vi "仁科遥控对话框.vi"() -> ()   [LabVIEW 2016, in "环境动力监测库.lvlib" / "空调库.lvlib"]
panel:
  in  "关机发射":bool
  in  "开机制热发射":bool
  in  "开机制冷发射":bool
  in  "关机学习":bool
  in  "开机制热学习":bool
  in  "开机制冷学习":bool
  # "学习遥控器"
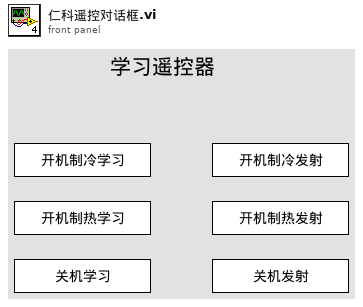
[diagram p1: front panel]
types:
  T1 = enum16{"open", "read", "write single", "write", "close"}
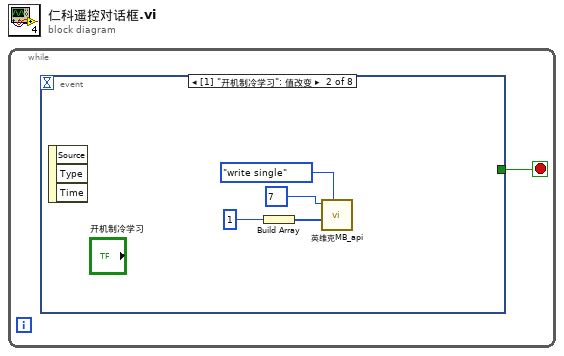
[diagram p0: block diagram]
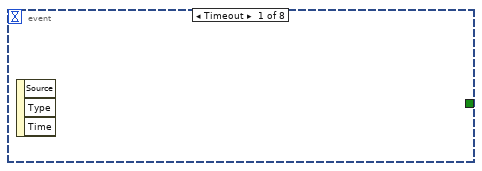
[diagram p2: hidden frame]
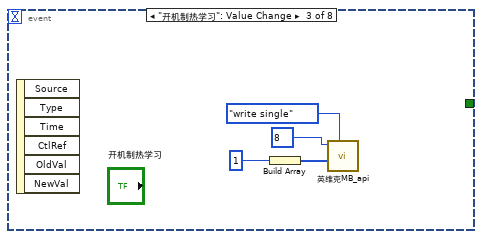
[diagram p3: hidden frame]
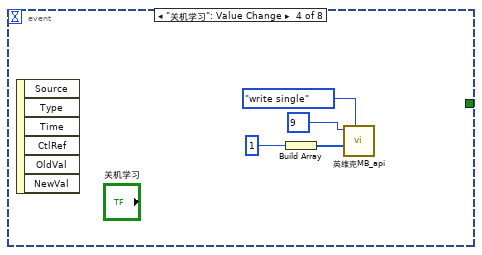
[diagram p4: hidden frame]
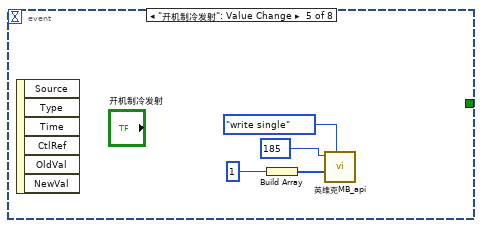
[diagram p5: hidden frame]
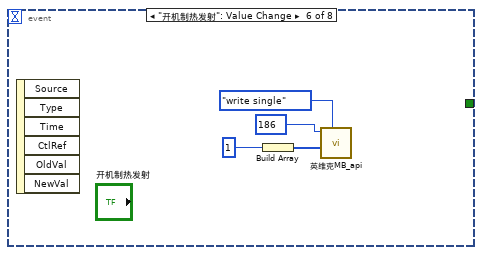
[diagram p6: hidden frame]
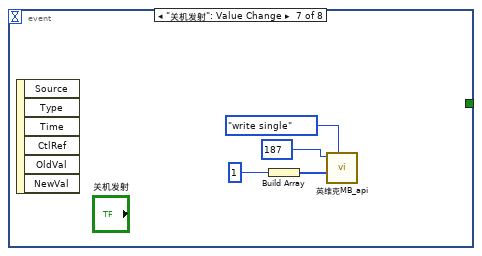
[diagram p7: hidden frame]
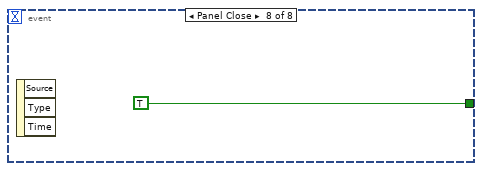
[diagram p8: hidden frame]
diagram:
  n1 = while {
    stop <- w1 stop-if-true
    n2 = event shown="[1] \"开机制冷学习\": 值改变" {
      selector: _ -> [_ _ _ _ _ _ _ _]
      dyn-events: _ -> [_ _ _ _ _ _ _ _]
      timeout: _ -> [_ _ _ _ _ _ _ _]
      tunnel: [_ _ _ _ _ _ _ TRUE] -> w1
      event Timeout {
        n3 = event-data() -> ()  [unwired: 1 in, 3 out]
      }
      event "开机制冷学习": Value Change {
        n4 = event-data() -> ()  [unwired: 1 in, 3 out]
        n5 = Build Array(u16 1) -> (w4:u16[])
        n6 = call "英维克MB_api.vi"("STEP"=T1."write single", "values"=w4, "starting address"=u16 7) -> ()  [unwired: 6 in, 3 out]
      }
      event "开机制热学习": Value Change {
        n7 = event-data() -> ()  [unwired: 1 in, 6 out]
        n8 = Build Array(u16 1) -> (w8:u16[])
        n9 = call "英维克MB_api.vi"("STEP"=T1."write single", "values"=w8, "starting address"=u16 8) -> ()  [unwired: 6 in, 3 out]
      }
      event "关机学习": Value Change {
        n10 = event-data() -> ()  [unwired: 1 in, 6 out]
        n11 = Build Array(u16 1) -> (w12:u16[])
        n12 = call "英维克MB_api.vi"("STEP"=T1."write single", "values"=w12, "starting address"=u16 9) -> ()  [unwired: 6 in, 3 out]
      }
      event "开机制冷发射": Value Change {
        n13 = event-data() -> ()  [unwired: 1 in, 6 out]
        n14 = Build Array(u16 1) -> (w16:u16[])
        n15 = call "英维克MB_api.vi"("STEP"=T1."write single", "values"=w16, "starting address"=u16 185) -> ()  [unwired: 6 in, 3 out]
      }
      event "开机制热发射": Value Change {
        n16 = event-data() -> ()  [unwired: 1 in, 6 out]
        n17 = Build Array(u16 1) -> (w20:u16[])
        n18 = call "英维克MB_api.vi"("STEP"=T1."write single", "values"=w20, "starting address"=u16 186) -> ()  [unwired: 6 in, 3 out]
      }
      event "关机发射": Value Change {
        n19 = event-data() -> ()  [unwired: 1 in, 6 out]
        n20 = Build Array(u16 1) -> (w24:u16[])
        n21 = call "英维克MB_api.vi"("STEP"=T1."write single", "values"=w24, "starting address"=u16 187) -> ()  [unwired: 6 in, 3 out]
      }
      event Panel Close {
        n22 = event-data() -> ()  [unwired: 1 in, 3 out]
      }
    }
  }
